vi "Self Event Alias.vi"(11 "Base Event jettl in":refnum<class "Base Event jettl.lvclass">) -> (2 "Self Event Alias":string)   [LabVIEW 2021, in "jettl.lvlib" / "Base Event jettl.lvlib" / "Base Event jettl.lvclass"]
uses:
  Base Event jettl.lvclass
  Base Event jettl.lvclass/Base Event jettl.ctl
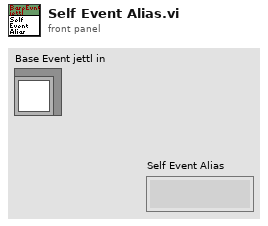
[diagram p1: front panel]
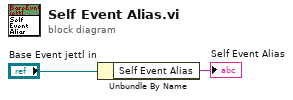
[diagram p0: block diagram]
diagram:
  n1 = Unbundle By Name("Base Event jettl in") -> ("Self Event Alias"=→"Self Event Alias":string)
